vi "byte-oscilloscope.vi"() -> ()   [LabVIEW 2023]
uses:
  <vilib>/Analysis/2dsp.llb/Decimate (single shot, DBL).vi
  <vilib>/Instr/_visa.llb/VISA Configure Serial Port (Instr).vi
  <vilib>/express/express analysis/Spectral/Block/exnSpectralBlock spectral measurements peak poly.vi
  <vilib>/express/express analysis/Spectral/Block/exnSpectralBlock spectral measurements peak WFM.vi
  <vilib>/express/express analysis/Spectral/XNode/ExpressSpectralMeasurementsBlockNode.xnode
  <vilib>/Analysis/NI_AALPro.lvlib
panel:
  out "Sampling Period (s)":sgl
  in  "Reference Voltage (V)":sgl
  in  "Baud Rate (BPS)":u32=9600
  in  "COM Port":refnum<visa-resource-name>
  in  "Stop Button":bool
  out "Time Domain":waveform(dbl)(graph)
  out "Frequency Domain":cluster{"f0":dbl, "df":dbl, "magnitude":dbl[]}(graph)
  in  "Time Domain (Block Size)":u16(knob) scale=4.0..10.0
  in  "Frequency Domain (Block Size)":u16(knob) scale=4.0..10.0
  out "Frerquency Domain Indicator":u32
  out "Time Domain Indicator":u32
  in  "Sampling Frequency (Hz)":sgl
  in  "Refresh Button":bool
  in  "Decimation Factor":u8=1 min=1 max=100
  # "BYTE-OSCILOSCOPE"
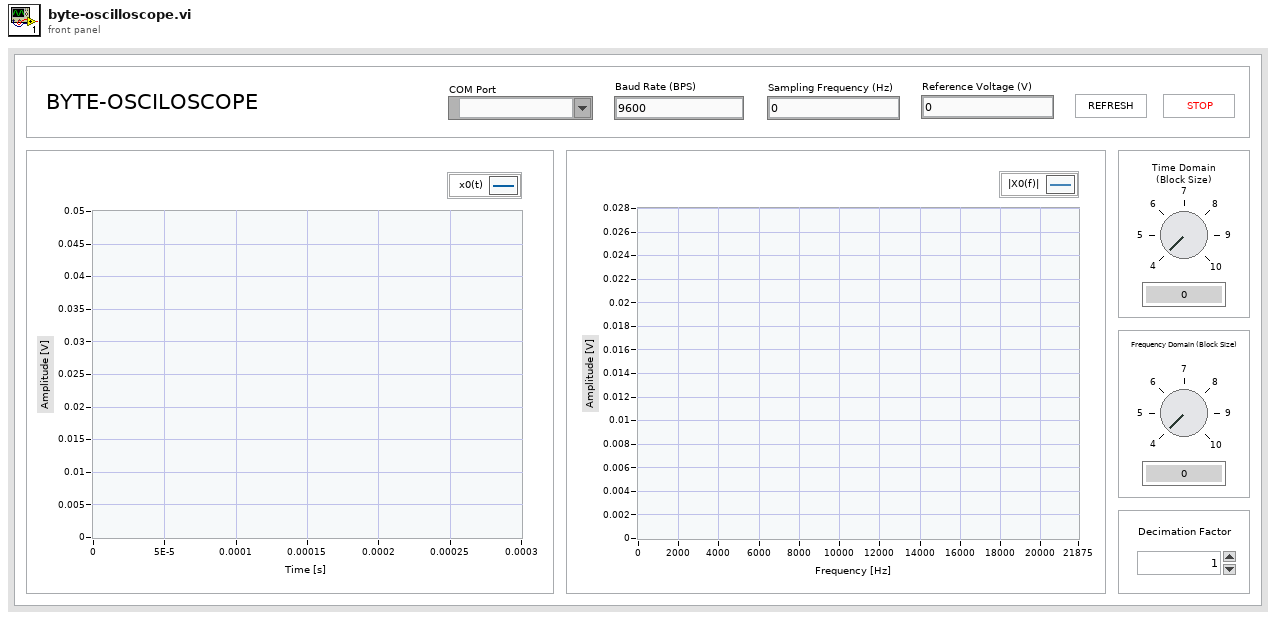
[diagram p1: front panel]
types:
  T1 = cluster{"averaging mode":u16, "weighting mode":u16, "number of averages":u32}
  T2 = cluster{"dB On (F)":bool, "unwrap phase (F)":bool, "convert to degree (F)":bool}
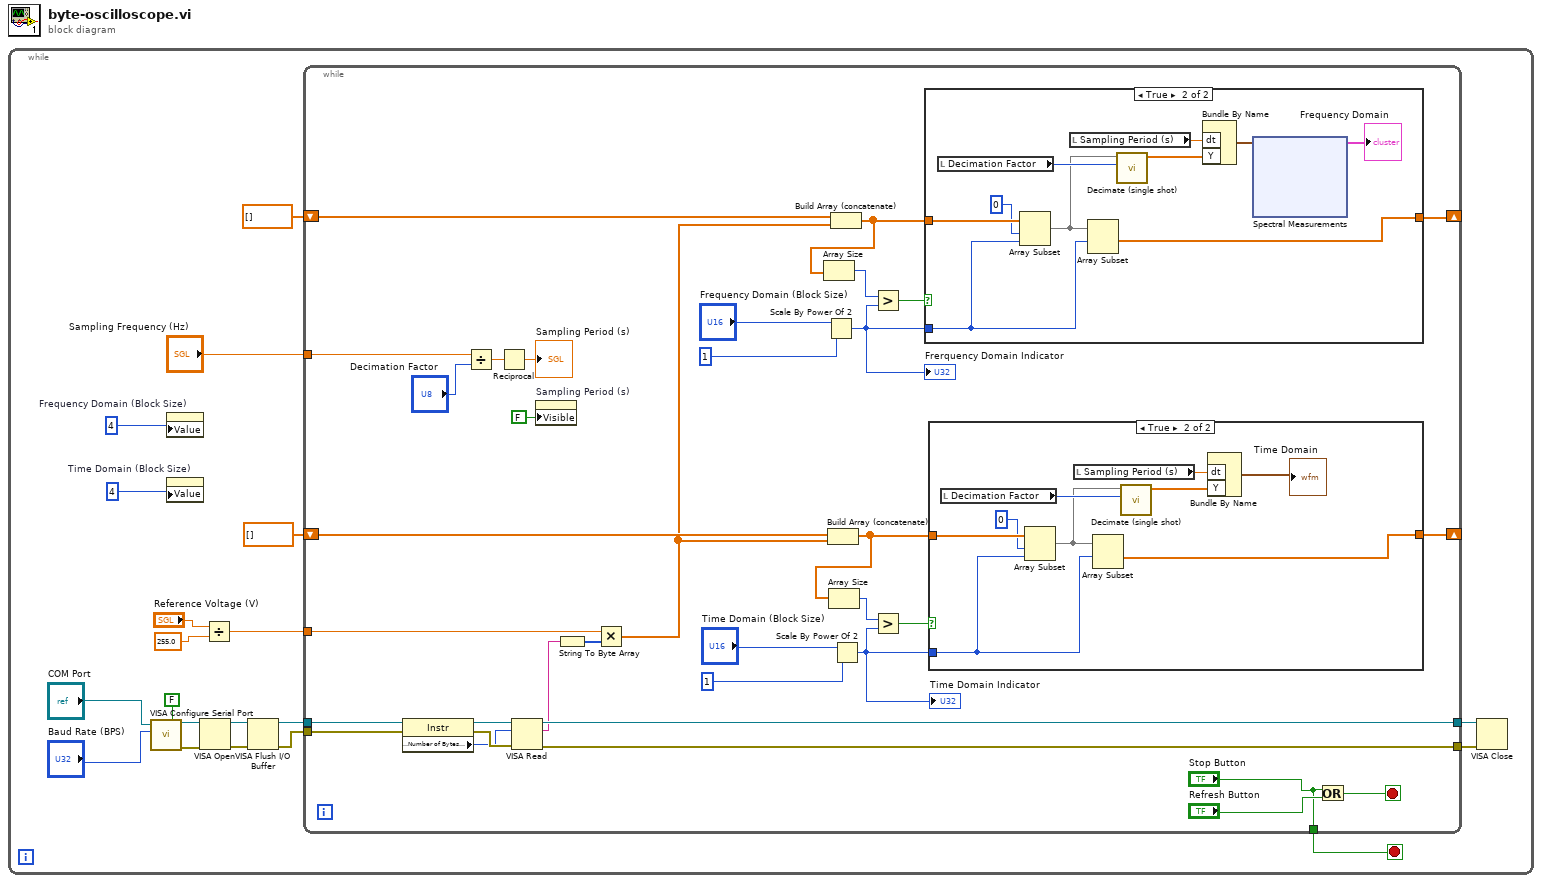
[diagram p0: block diagram]
diagram:
  n1 = while {
    stop <- w10 stop-if-true
    n2 = call-poly "VISA Configure Serial Port"("VISA resource name"="COM Port", "Enable Termination\nChar (T)"=FALSE ("Enable Termination\nChar (T)"), "baud rate (9600)"="Baud Rate (BPS)") -> ("VISA resource name out"=w18:refnum<visa-resource-name>, "error out"=w19:errorcluster)  [unwired: 11 in]
    n3 = property on="Frequency Domain (Block Size)" class="Knob (strict)"("Value"=u16 4 ("Frequency Domain (Block Size)")) -> ()  [unwired: 2 in, 2 out]
    n4 = property on="Time Domain (Block Size)" class="Knob (strict)"("Value"=u16 4 ("Time Domain (Block Size)")) -> ()  [unwired: 2 in, 2 out]
    n5 = VISA Open(error in (no error)=w19, VISA resource name=w18) -> (VISA resource name=w17:refnum<visa-resource-name>, error out=w16:errorcluster)  [unwired: 3 in]
    n6 = Divide(x="Reference Voltage (V)", y=255.0) -> (x/y=w2:dbl)
    n7 = VISA Flush I/O Buffer(VISA resource name=w17, error in (no error)=w16) -> (VISA resource name out=w20:refnum<visa-resource-name>, error out=w15:errorcluster)  [unwired: 1 in]
    n8 = while {
      tunnel: w20 -> [w55]
      tunnel: w15 -> [w54]
      tunnel: [w47] -> w14
      tunnel: [w48] -> w13
      shift-right: [w49] -> _
      shift-left: dbl[] [] -> [w50]
      shift-right: [w45] -> _
      shift-left: dbl[] [] -> [w46]
      tunnel: ["Stop Button"] -> w10
      tunnel: w2 -> [w22]
      tunnel: "Sampling Frequency (Hz)" -> [w21]
      stop <- w44 stop-if-true
      n9 = property class="Instr"(reference=w55, error in=w54) -> (reference out=w53:refnum<visa-resource-name>, error out=w52:errorcluster, "Serial Settings:Number of Bytes at Serial Port"=w51:u32)
      n10 = Divide(x=w21, y="Decimation Factor") -> (x/y=w27:sgl)
      n11 = Reciprocal(x=w27) -> (1/x=→"Sampling Period (s)":sgl)
      n12 = VISA Read(VISA resource name=w53, byte count=w51, error in (no error)=w52) -> (VISA resource name out=w48:refnum<visa-resource-name>, read buffer=w29:string, error out=w47:errorcluster)  [unwired: 1 out]
      n13 = property on="Sampling Period (s)" class="DigNum (strict)"("Visible"=FALSE) -> ()  [unwired: 2 in, 2 out]
      n14 = String To Byte Array(string=w29) -> (unsigned byte array=w23:u8[])
      n15 = Multiply(x=w22, y=w23) -> (x*y=w24:dbl[])
      n16 = Scale By Power Of 2(n="Frequency Domain (Block Size)", x=u32 1) -> (x*2^n=w33:u32)
      "Frerquency Domain Indicator" <- w33
      n17 = Build Array (concatenate)(w50, w24) -> (w34:dbl[])
      n18 = Array Size(array=w34) -> (size(s)=w41:i32)
      n19 = Build Array (concatenate)(w46, w24) -> (w35:dbl[])
      n20 = Array Size(array=w35) -> (size(s)=w38:i32)
      n21 = Scale By Power Of 2(n="Time Domain (Block Size)", x=u32 1) -> (x*2^n=w32:u32)
      "Time Domain Indicator" <- w32
      n22 = Greater?(x=w38, y=w33) -> (0:w39:bool)
      n23 = Greater?(x=w41, y=w32) -> (0:w40:bool)
      n24 = case shown="True" w39 {
        tunnel: w35 -> [w56 w66]
        tunnel: [w56 w64] -> w45
        tunnel: w33 -> [_ w62]
        frame False {
        }
        frame True {
          n25 = local read "Decimation Factor"() -> (w59:u8)
          n26 = Array Subset(array=w66, index=0, length=w62) -> (w58:dbl[])
          n27 = local read "Sampling Period (s)"() -> (w60:sgl)
          n28 = Array Subset(array=w58, index=w62) -> (w64:dbl[])  [unwired: 1 in]
          n29 = call-poly <vilib>:"Decimate (single shot).vi"("decimating factor"=w59, "X"=w58) -> ("Decimated Array"=w57:dbl[])  [unwired: 8 in, 1 out]
          n30 = Bundle By Name("dt"=w60, "Y"=w57) -> (w63:waveform(dbl))  [unwired: 1 in]
          n31 = xnode "Spectral Measurements"("Signals"=w63) -> ("FFT - (Peak)"=→"Frequency Domain":cluster{"f0":dbl, "df":dbl, "magnitude":dbl[]})  [unwired: 1 in, 2 out]
        }
      }
      n32 = case shown="True" w40 {
        tunnel: w34 -> [w77 w86]
        tunnel: w32 -> [_ w85]
        tunnel: [w77 w84] -> w49
        frame False {
        }
        frame True {
          n33 = local read "Decimation Factor"() -> (w80:u8)
          n34 = Array Subset(array=w86, index=0, length=w85) -> (w79:dbl[])
          n35 = local read "Sampling Period (s)"() -> (w81:sgl)
          n36 = Array Subset(array=w79, index=w85) -> (w84:dbl[])  [unwired: 1 in]
          n37 = call-poly <vilib>:"Decimate (single shot).vi"("decimating factor"=w80, "X"=w79) -> ("Decimated Array"=w78:dbl[])  [unwired: 8 in, 1 out]
          n38 = Bundle By Name("dt"=w81, "Y"=w78) -> (→"Time Domain":waveform(dbl))  [unwired: 1 in]
        }
      }
      n39 = Or(x="Stop Button", y="Refresh Button") -> (x .or. y?=w44:bool)
    }
    n40 = VISA Close(VISA resource name=w13, error in (no error)=w14) -> ()  [unwired: 1 out]
  }
